vi "Get Server Type and Status.vi"(0 "All Interfaces Dict":variant, 2 "Specific Interface Dict in":variant, 3 "Listener Settings":T1, 5 "error in (no error)":errorcluster) -> (14 "Is \"All Interface\" Server":bool, 15 "Server Running":bool, 16 "Server URI":string, 19 "error out":errorcluster)   [LabVIEW 2016, in "WebSocket Actors.lvlib" / "WebSocket Server Manager.lvclass"]
uses:
  WebSocket Server Manager.lvclass
  WebSocket Server/typedefs/Listener Settings.ctl
  WebSocket Server/WebSocket Server.lvclass
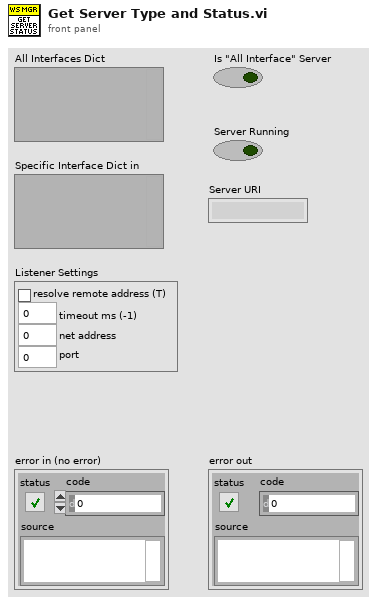
[diagram p1: front panel]
types:
  T1 = typedef "WebSocket Actors.lvlib/WebSocket Server.lvclass/Listener Settings.ctl" = cluster{"resolve remote address (T)":bool, "timeout ms (-1)":i32, "net address":u32, "port":u16}
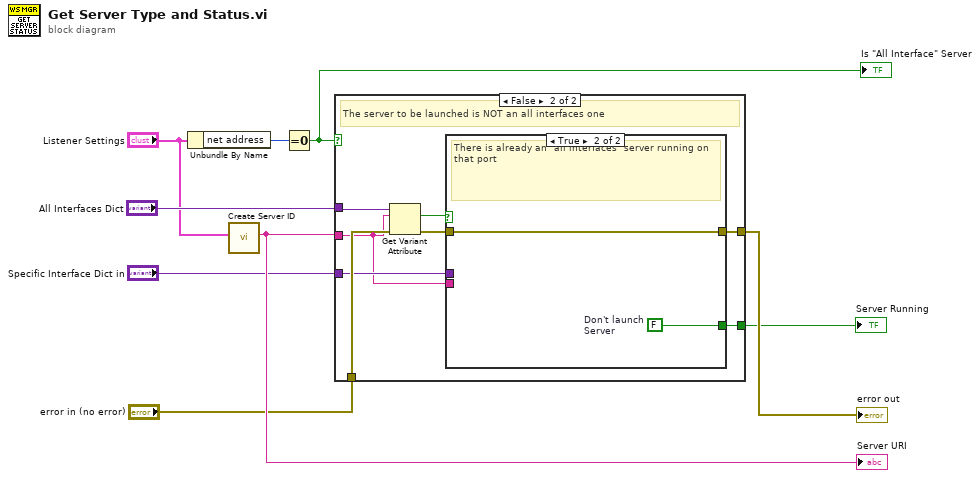
[diagram p0: block diagram]
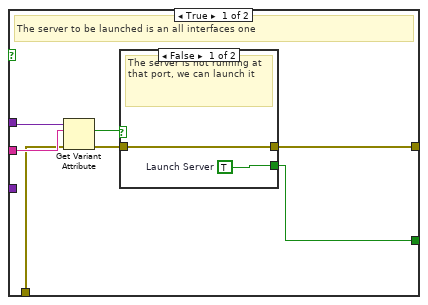
[diagram p2: hidden frame]
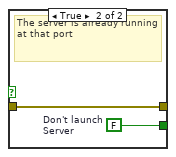
[diagram p3: hidden frame]
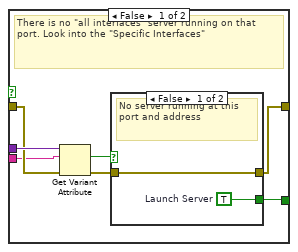
[diagram p4: hidden frame]
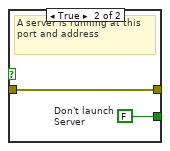
[diagram p5: hidden frame]
diagram:
  n1 = Unbundle By Name("Listener Settings") -> ("net address"=w2:u32)
  n2 = call "Create Server ID.vi"("Listener Settings"="Listener Settings") -> ("Server URI"=w8:string)  [unwired: 7 in, 2 out]
  "Server URI" <- w8
  n3 = Equal To 0?(x=w2) -> (x = 0?=w7:bool)
  "Is \"All Interface\" Server" <- w7
  n4 = case shown="False" w7 {
    tunnel: "Specific Interface Dict in" -> [_ w24]
    tunnel: "All Interfaces Dict" -> [w16 w28]
    tunnel: w8 -> [w14 w21]
    tunnel: "error in (no error)" -> [w13 w26]
    tunnel: [w11 w22] -> w9
    tunnel: [w10 w23] -> w6
    frame True {
      # "The server to be launched is an all interfaces one"
      n5 = Get Variant Attribute(Variant=w16, name=w14, error in=w13) -> (found=w15:bool, error out=w12:errorcluster)  [unwired: 1 in, 2 out]
      n6 = case shown="False" w15 {
        tunnel: w12 -> [w18 w19]
        tunnel: [w18 w19] -> w11
        tunnel: [w17 w20] -> w10
        frame False {
          w17 = TRUE  # Launch Server
          # "The server is not running at that port, we can launch it"
        }
        frame True {
          w20 = FALSE  # Don't launch  Server
          # "The server is already running at that port"
        }
      }
    }
    frame False {
      # "The server to be launched is NOT an all interfaces one"
      n7 = Get Variant Attribute(Variant=w28, name=w21, error in=w26) -> (found=w27:bool, error out=w25:errorcluster)  [unwired: 1 in, 2 out]
      n8 = case shown="True" w27 {
        tunnel: w25 -> [w34 w40]
        tunnel: [w29 w40] -> w22
        tunnel: [w30 w41] -> w23
        tunnel: w24 -> [w35 _]
        tunnel: w21 -> [w33 _]
        frame False {
          # "There is no \"all interfaces\" server running on that port. Look into the \"Specific Interfaces\""
          n9 = Get Variant Attribute(Variant=w35, name=w33, error in=w34) -> (found=w32:bool, error out=w31:errorcluster)  [unwired: 1 in, 2 out]
          n10 = case shown="False" w32 {
            tunnel: w31 -> [w36 w38]
            tunnel: [w37 w39] -> w30
            tunnel: [w36 w38] -> w29
            frame False {
              w37 = TRUE  # Launch Server
              # "No server running at this port and address"
            }
            frame True {
              w39 = FALSE  # Don't launch  Server
              # "A server is running at this port and address"
            }
          }
        }
        frame True {
          w41 = FALSE  # Don't launch  Server
          # "There is already an \"all interfaces\" server running on that port"
        }
      }
    }
  }
  "error out" <- w9
  "Server Running" <- w6
